vi "Set Wheel Motors Velocity Setpoint.vi"(8 "error in (no error)":errorcluster, 10 "ccw velocity (rad/s)":dbl[](array[numeric]), 11 "KUKA youBot platform in":refnum<class "NI_Robotics_KUKA youBot Platform.lvclass">) -> (0 "error out":errorcluster, 3 "KUKA youBot platform out":refnum<class "NI_Robotics_KUKA youBot Platform.lvclass">)   [LabVIEW 2017, in "NI_Robotics_KUKA youBot Host.lvlib" / "NI_Robotics_KUKA youBot Platform.lvclass"]
doc: "Sets the motors velocity setpoint of the wheels of a KUKA youBot mobile platform."
uses:
  <vilib>/robotics/KUKA youBot/Basic Device/Mobile Platform/NI_Robotics_KUKA youBot Platform.lvclass
  <vilib>/robotics/KUKA youBot/Basic Device/Mobile Platform/NI_Robotics_KUKA youBot Platform.lvclass/NI_Robotics_KUKA youBot Platform.ctl
  <vilib>/robotics/KUKA youBot/Motor/Wheel Motor/NI_Robotics_KUKA youBot Wheel Motor.lvclass
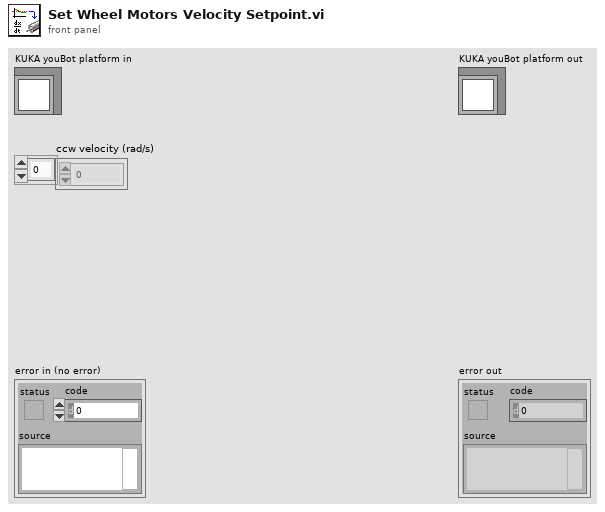
[diagram p1: front panel]
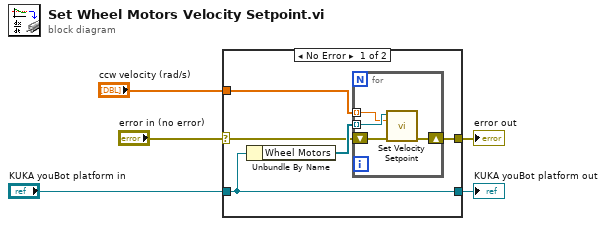
[diagram p0: block diagram]
diagram:
  n1 = case shown="No Error" "error in (no error)" {
    selector: "error in (no error)" -> [w8 w15]
    tunnel: [w7 w15] -> w4
    tunnel: [w6 w16] -> w2
    tunnel: "KUKA youBot platform in" -> [w6 w16]
    tunnel: "ccw velocity (rad/s)" -> [w9 _]
    frame No Error {
      n2 = Unbundle By Name(w6) -> ("Wheel Motors"=w10:refnum<class "NI_Robotics_KUKA youBot Wheel Motor.lvclass">[])
      n3 = for {
        tunnel: w10 -> [w14] mode=indexing
        tunnel: w9 -> [w13] mode=indexing
        shift-right: [w11] -> w7
        shift-left: w8 -> [w12]
        n4 = call-dynamic "Set Velocity Setpoint.vi"("error in (no error)"=w12, "CCW velocity (rad/s)"=w13, "KUKA youBot wheel motor in"=w14) -> ("error out"=w11:errorcluster)  [unwired: 7 in, 1 out]
      }
    }
    frame Error {
    }
  }
  "error out" <- w4
  "KUKA youBot platform out" <- w2
